vi "Get Fit Settings.vi"(6 "Fit Model":T2, 8 "Error In":errorcluster, 9 "Additional Parameters":variant, 10 "Fixed Parameters":T3, 11 "XY Graph Ref":refnum<vi>) -> (0 "Error Out":errorcluster, 1 "Fit Model Information":T1, 2 "Additional Fit Settings":variant, 3 "LM Function & Gradient":refnum<vi>)   [LabVIEW 2021, in "Fits.lvlib"]
uses:
  Fits.lvlib
  Fit Models.ctl
  D-Only Fixed Parameters.ctl
  N Components Additional Fit Settings.ctl
  Gaussian/LM Gaussian and gradient.vi
  Asymmetric Gaussian/LM Asymmetric Gaussian and gradient.vi
  Lorentzian/LM Lorentzian and gradient.vi
  Asymmetric Lorentzian/LM Asymmetric Lorentzian and gradient.vi
  Gaussian-Lorentzian/LM Gaussian-Lorentzian and gradient.vi
  Lorentzian-Gaussian/LM Lorentzian-Gaussian and gradient.vi
  Two Gaussians/LM Two Gaussians and gradient.vi
  Two Asymmetric Gaussians/LM Two Asymmetric Gaussians and gradient.vi
  Two Connected Asymmetric Gaussians/LM Two H-Connected Asymmetric Gaussians and gradient.vi
  Two Connected Asymmetric Gaussians/LM Two T-Connected Asymmetric Gaussians and gradient.vi
  Two Connected Gaussians/LM Two H-Connected Gaussians and gradient.vi
  Two Connected Gaussians/LM Two T-Connected Gaussians and gradient.vi
  Three Gaussians/LM Three Gaussians and gradient.vi
  Three Asymmetric Gaussians/LM Three Asymmetric Gaussians and gradient.vi
  Single Exponential/LM Single Exponential and gradient.vi
  IRF(X)PSED/LM IRF(X)PSED and gradient v4.vi
  Double Exponential/LM Double Exponential and gradient.vi
  Power Law/LM Power Law with Offset and gradient.vi
  Power Law/LM Power Law and gradient.vi
  ACF-CCF/2D ACF/LM 2D Gaussian ACF and gradient.vi
  ACF-CCF/2D ACF/LM 2D Gaussian + Blinking ACF and gradient.vi
  ACF-CCF/2D ACF/LM 2D Gaussian + Flow ACF and gradient.vi
  ACF-CCF/3D ACF/LM 3D Gaussian ACF and gradient.vi
  ACF-CCF/3D ACF/LM 3D Gaussian + Blinking ACF and gradient.vi
  ACF-CCF/2D ACF/LM 2D Gaussian ACF + Flow and gradient (Global).vi
  Variant/Variant to Data/Variant to I32.vi
  Variant/Variant to Data/Variant to Data.lvlib
  Fit Model Information.ctl
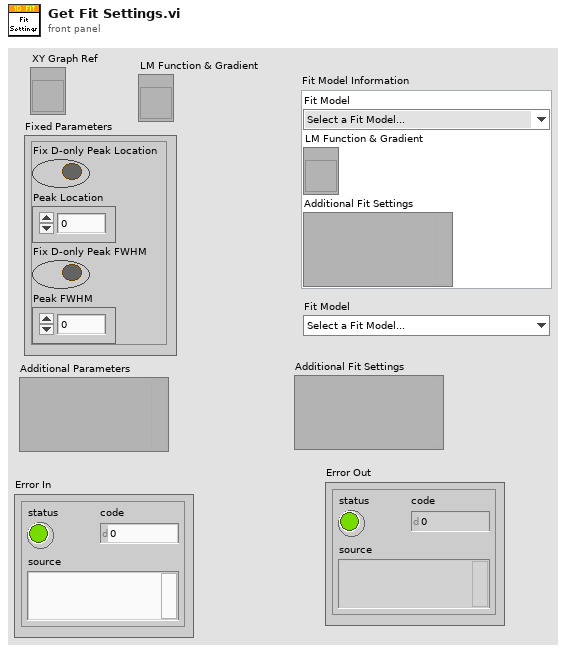
[diagram p1: front panel]
types:
  T1 = typedef "Fits.lvlib/Fit Model Information.ctl" = cluster{"Fit Model":T2, "LM Function & Gradient":refnum<vi>, "Additional Fit Settings":variant}
  T2 = typedef "Fits.lvlib/Fit Models.ctl" = enum16{"Select a Fit Model...", "           Single Peak", "Gaussian", "Asymmetric Gaussian", "Lorentzian", "Asymmetric Lorentzian", "Gaussian/Lorentzian", "Lorentzian/Gaussian", "           Double Peak", "Two Gaussians", "Two Asymmetric Gaussians", "Two H-Connected Gaussians", "Two T-Connected Gaussians", "Two H-Connected Asymmetric Gaussians", "Two T-Connected Asymmetric Gaussians", "           Triple Peak", "Three Gaussians", "Three Asymmetric Gaussians", "              Decays", "1-Exponential", "IRF*PSED", "2-Exponentials", "            Power Law", "Power Law", "Power Law with Offset", "               ACF", "2D Gaussian ACF", "2D Gaussian + Blinking ACF", "2D Gaussian + Flow ACF", "3D Gaussian ACF", "3D Gaussian + Blinking ACF", "             Multiplot", "2D Gaussian ACF & 2D Gaussian + Flow ACF"}
  T3 = typedef "Fits.lvlib/D-Only Fixed Parameters.ctl" = cluster{"Fix D-only Peak Location":bool, "Peak Location":dbl, "Fix D-only Peak FWHM":bool, "Peak FWHM":dbl}
  T4 = typedef "Fits.lvlib/N Components Additional Fit Settings.ctl" = cluster{"Fixed Parameters":T3, "Cursor Coordinates":dbl[], "Data Split Point":i32}
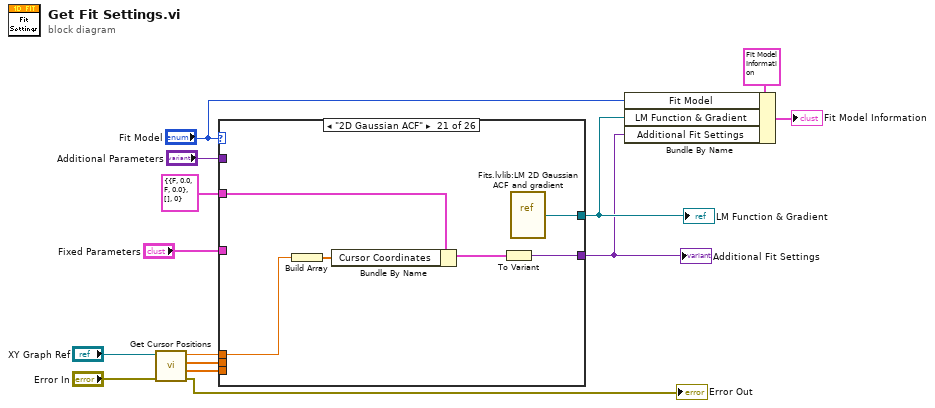
[diagram p0: block diagram]
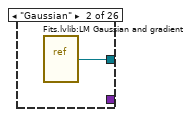
[diagram p3: hidden frame]
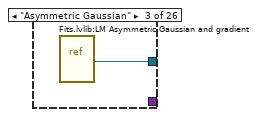
[diagram p4: hidden frame]
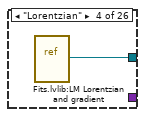
[diagram p5: hidden frame]
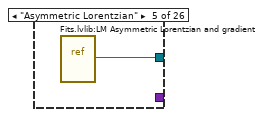
[diagram p6: hidden frame]
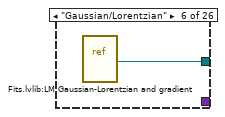
[diagram p7: hidden frame]
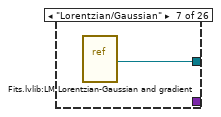
[diagram p8: hidden frame]
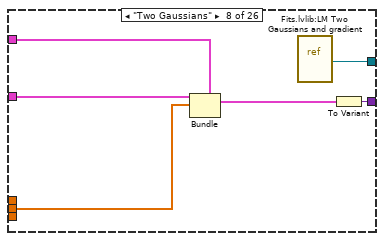
[diagram p9: hidden frame]
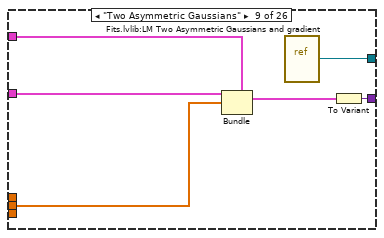
[diagram p10: hidden frame]
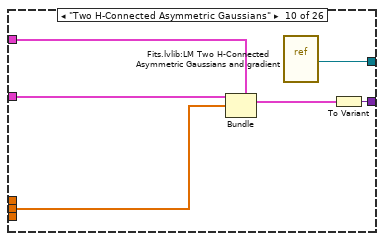
[diagram p11: hidden frame]
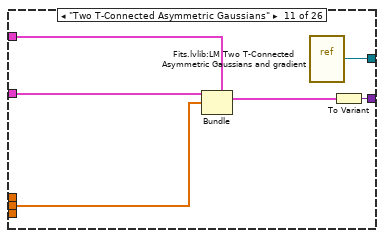
[diagram p12: hidden frame]
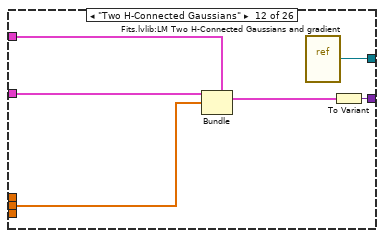
[diagram p13: hidden frame]
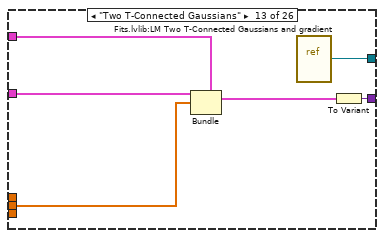
[diagram p14: hidden frame]
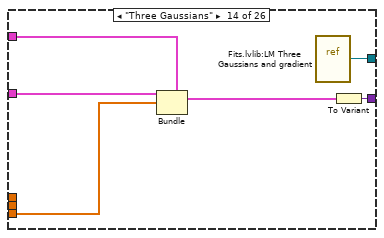
[diagram p15: hidden frame]
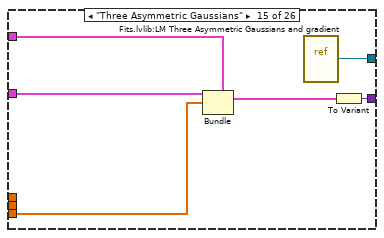
[diagram p16: hidden frame]
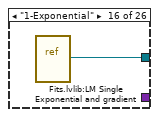
[diagram p17: hidden frame]
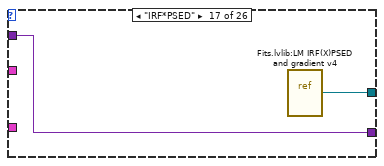
[diagram p18: hidden frame]
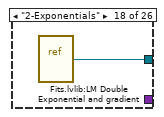
[diagram p19: hidden frame]
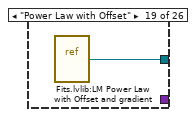
[diagram p20: hidden frame]
diagram:
  n1 = call "Get Cursor Positions.vi"("Error In"="Error In", "XYGraph in"="XY Graph Ref") -> ("Error Out"=→"Error Out":errorcluster, "Cursor 1-3 Positions"=w10:dbl[], "Cursor 1 & 2 Positions"=w11:dbl[], "Cursor 1 Position"=w12:dbl)  [unwired: 6 in]
  n2 = case shown="\"2D Gaussian ACF\"" "Fit Model" {
    tunnel: "Fixed Parameters" -> [_ _ _ _ _ _ _ w26 w32 w38 w44 w50 w56 w62 w68 _ _ _ _ _ _ _ _ _ _ _]
    tunnel: [_ _ _ _ _ _ _ w24 w30 w36 w42 w48 w54 w60 w66 _ w70 _ _ _ w75 w81 w86 w91 w97 w102] -> w1
    tunnel: w10 -> [_ _ _ _ _ _ _ _ _ _ _ _ _ w59 w65 _ _ _ _ _ _ _ _ _ _ _]
    tunnel: w11 -> [_ _ _ _ _ _ _ w23 w29 w35 w41 w47 w53 _ _ _ _ _ _ _ _ w84 w89 _ w100 w104]
    tunnel: w12 -> [_ _ _ _ _ _ _ _ _ _ _ _ _ _ _ _ _ _ _ _ w80 _ _ w96 _ _]
    tunnel: T4 {"Fixed Parameters"={"Fix D-only Peak Location"=FALSE, "Peak Location"=0.0, "Fix D-only Peak FWHM"=FALSE, "Peak FWHM"=0.0}, "Cursor Coordinates"=[], "Data Split Point"=0} ("N Components Additional Fit Settings") -> [_ _ _ _ _ _ _ w22 w28 w34 w40 w46 w52 w58 w64 _ _ _ _ _ w77 w83 w88 w93 w99 w108]
    tunnel: "Additional Parameters" -> [_ _ _ _ _ _ _ _ _ _ _ _ _ _ _ _ w70 _ _ _ _ _ _ _ _ w106]
    tunnel: [_ w15 w16 w17 w18 w19 w20 w21 w27 w33 w39 w45 w51 w57 w63 w69 w71 w72 w73 w74 w76 w82 w87 w92 w98 w103] -> w2
    frame "Select a Fit Model...", Default {
    }
    frame "Gaussian" {
      n3 = vi-ref "Fits.lvlib:LM Gaussian and gradient.vi"() -> (w15:refnum<vi>)
    }
    frame "Asymmetric Gaussian" {
      n4 = vi-ref "Fits.lvlib:LM Asymmetric Gaussian and gradient.vi"() -> (w16:refnum<vi>)
    }
    frame "Lorentzian" {
      n5 = vi-ref "Fits.lvlib:LM Lorentzian and gradient.vi"() -> (w17:refnum<vi>)
    }
    frame "Asymmetric Lorentzian" {
      n6 = vi-ref "Fits.lvlib:LM Asymmetric Lorentzian and gradient.vi"() -> (w18:refnum<vi>)
    }
    frame "Gaussian/Lorentzian" {
      n7 = vi-ref "Fits.lvlib:LM Gaussian-Lorentzian and gradient.vi"() -> (w19:refnum<vi>)
    }
    frame "Lorentzian/Gaussian" {
      n8 = vi-ref "Fits.lvlib:LM Lorentzian-Gaussian and gradient.vi"() -> (w20:refnum<vi>)
    }
    frame "Two Gaussians" {
      n9 = Bundle(cluster=w22, "Fixed Parameters"=w26, "Cursor Coordinates"=w23) -> (w25:T4)  [unwired: 1 in]
      n10 = vi-ref "Fits.lvlib:LM Two Gaussians and gradient.vi"() -> (w21:refnum<vi>)
      n11 = To Variant(anything=w25) -> (Variant=w24:variant)
    }
    frame "Two Asymmetric Gaussians" {
      n12 = Bundle(cluster=w28, "Fixed Parameters"=w32, "Cursor Coordinates"=w29) -> (w31:T4)  [unwired: 1 in]
      n13 = vi-ref "Fits.lvlib:LM Two Asymmetric Gaussians and gradient.vi"() -> (w27:refnum<vi>)
      n14 = To Variant(anything=w31) -> (Variant=w30:variant)
    }
    frame "Two H-Connected Asymmetric Gaussians" {
      n15 = Bundle(cluster=w34, "Fixed Parameters"=w38, "Cursor Coordinates"=w35) -> (w37:T4)  [unwired: 1 in]
      n16 = vi-ref "Fits.lvlib:LM Two H-Connected Asymmetric Gaussians and gradient.vi"() -> (w33:refnum<vi>)
      n17 = To Variant(anything=w37) -> (Variant=w36:variant)
    }
    frame "Two T-Connected Asymmetric Gaussians" {
      n18 = Bundle(cluster=w40, "Fixed Parameters"=w44, "Cursor Coordinates"=w41) -> (w43:T4)  [unwired: 1 in]
      n19 = vi-ref "Fits.lvlib:LM Two T-Connected Asymmetric Gaussians and gradient.vi"() -> (w39:refnum<vi>)
      n20 = To Variant(anything=w43) -> (Variant=w42:variant)
    }
    frame "Two H-Connected Gaussians" {
      n21 = Bundle(cluster=w46, "Fixed Parameters"=w50, "Cursor Coordinates"=w47) -> (w49:T4)  [unwired: 1 in]
      n22 = vi-ref "Fits.lvlib:LM Two H-Connected Gaussians and gradient.vi"() -> (w45:refnum<vi>)
      n23 = To Variant(anything=w49) -> (Variant=w48:variant)
    }
    frame "Two T-Connected Gaussians" {
      n24 = Bundle(cluster=w52, "Fixed Parameters"=w56, "Cursor Coordinates"=w53) -> (w55:T4)  [unwired: 1 in]
      n25 = vi-ref "Fits.lvlib:LM Two T-Connected Gaussians and gradient.vi"() -> (w51:refnum<vi>)
      n26 = To Variant(anything=w55) -> (Variant=w54:variant)
    }
    frame "Three Gaussians" {
      n27 = Bundle(cluster=w58, "Fixed Parameters"=w62, "Cursor Coordinates"=w59) -> (w61:T4)  [unwired: 1 in]
      n28 = vi-ref "Fits.lvlib:LM Three Gaussians and gradient.vi"() -> (w57:refnum<vi>)
      n29 = To Variant(anything=w61) -> (Variant=w60:variant)
    }
    frame "Three Asymmetric Gaussians" {
      n30 = Bundle(cluster=w64, "Fixed Parameters"=w68, "Cursor Coordinates"=w65) -> (w67:T4)  [unwired: 1 in]
      n31 = vi-ref "Fits.lvlib:LM Three Asymmetric Gaussians and gradient.vi"() -> (w63:refnum<vi>)
      n32 = To Variant(anything=w67) -> (Variant=w66:variant)
    }
    frame "1-Exponential" {
      n33 = vi-ref "Fits.lvlib:LM Single Exponential and gradient.vi"() -> (w69:refnum<vi>)
    }
    frame "IRF*PSED" {
      n34 = vi-ref "Fits.lvlib:LM IRF(X)PSED and gradient v4.vi"() -> (w71:refnum<vi>)
    }
    frame "2-Exponentials" {
      n35 = vi-ref "Fits.lvlib:LM Double Exponential and gradient.vi"() -> (w72:refnum<vi>)
    }
    frame "Power Law with Offset" {
      n36 = vi-ref "Fits.lvlib:LM Power Law with Offset and gradient.vi"() -> (w73:refnum<vi>)
    }
    frame "Power Law" {
      n37 = vi-ref "Fits.lvlib:LM Power Law and gradient.vi"() -> (w74:refnum<vi>)
    }
    frame "2D Gaussian ACF" {
      n38 = Build Array(w80) -> (w79:dbl[])
      n39 = Bundle By Name(cluster=w77, "Cursor Coordinates"=w79) -> (w78:T4)
      n40 = To Variant(anything=w78) -> (Variant=w75:variant)
      n41 = vi-ref "Fits.lvlib:LM 2D Gaussian ACF and gradient.vi"() -> (w76:refnum<vi>)
    }
    frame "2D Gaussian + Blinking ACF" {
      n42 = Bundle By Name(cluster=w83, "Cursor Coordinates"=w84) -> (w85:T4)
      n43 = To Variant(anything=w85) -> (Variant=w81:variant)
      n44 = vi-ref "Fits.lvlib:LM 2D Gaussian + Blinking ACF and gradient.vi"() -> (w82:refnum<vi>)
    }
    frame "2D Gaussian + Flow ACF" {
      n45 = Bundle By Name(cluster=w88, "Cursor Coordinates"=w89) -> (w90:T4)
      n46 = To Variant(anything=w90) -> (Variant=w86:variant)
      n47 = vi-ref "Fits.lvlib:LM 2D Gaussian + Flow ACF and gradient.vi"() -> (w87:refnum<vi>)
    }
    frame "3D Gaussian ACF" {
      n48 = Build Array(w96) -> (w95:dbl[])
      n49 = Bundle By Name(cluster=w93, "Cursor Coordinates"=w95) -> (w94:T4)
      n50 = To Variant(anything=w94) -> (Variant=w91:variant)
      n51 = vi-ref "Fits.lvlib:LM 3D Gaussian ACF and gradient.vi"() -> (w92:refnum<vi>)
    }
    frame "3D Gaussian + Blinking ACF" {
      n52 = Bundle By Name(cluster=w99, "Cursor Coordinates"=w100) -> (w101:T4)
      n53 = To Variant(anything=w101) -> (Variant=w97:variant)
      n54 = vi-ref "Fits.lvlib:LM 3D Gaussian + Blinking ACF and gradient.vi"() -> (w98:refnum<vi>)
    }
    frame "2D Gaussian ACF & 2D Gaussian + Flow ACF" {
      n55 = call-poly "Variant to Data.vi"("Variant"=w106) -> ("Value"=w105:i32)  [unwired: 8 in]
      n56 = Bundle By Name(cluster=w108, "Data Split Point"=w105, "Cursor Coordinates"=w104) -> (w107:T4)
      n57 = vi-ref "Fits.lvlib:LM 2D Gaussian ACF + Flow and gradient (Global).vi"() -> (w103:refnum<vi>)
      n58 = To Variant(anything=w107) -> (Variant=w102:variant)
    }
  }
  "Additional Fit Settings" <- w1
  "LM Function & Gradient" <- w2
  n59 = Bundle By Name(cluster=T1 {"Fit Model"=enum."Select a Fit Model...", "LM Function & Gradient"=refnum, "Additional Fit Settings"=variant} ("Fit Model Information"), "Fit Model"="Fit Model", "LM Function & Gradient"=w2, "Additional Fit Settings"=w1) -> (→"Fit Model Information":T1)
